vi "main.vi"() -> ()   [LabVIEW 2019]
uses:
  <vilib>/userDefined/High Color/IMAQdx.ctl
  <vilib>/vision/Image Controls.llb/IMAQ Image.ctl
  <vilib>/vision/driver/NI_Vision_Acquisition_Software.lvlib
panel:
  in  "Tab Control":enum32{"Learn Pattern"}(tab)
  in  "Learn":bool
  out "Grab Image Duration":u32
  out "Stop Threads":bool
  out "Grab Running":bool
  out "Image Raw":T1
  out "error out":errorcluster
  in  "Session In":T2
  in  "Snap":bool
  in  "Stop":bool
  in  "Grab":bool
  out "Image Viewer":T1(plugin-control)
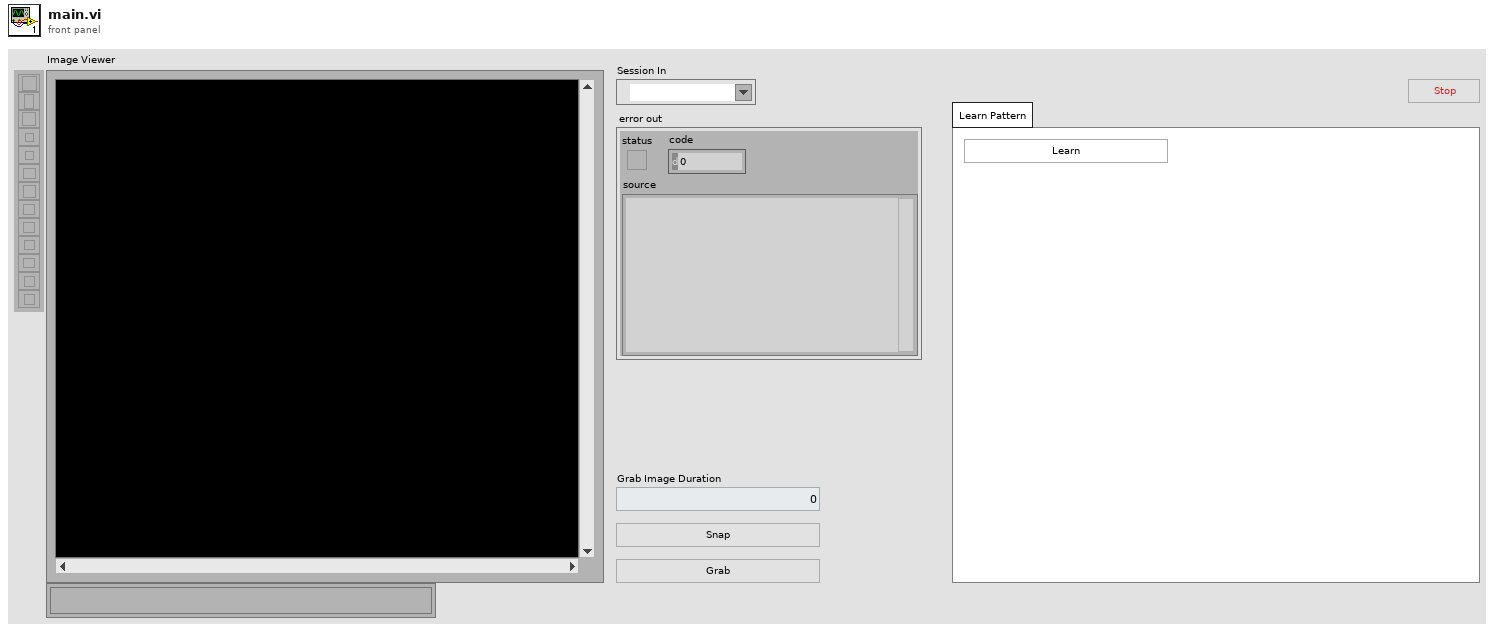
[diagram p1: front panel]
types:
  T1 = typedef "IMAQ Image.ctl" = refnum<image>
  T2 = typedef "IMAQdx.ctl" = refnum<k21>
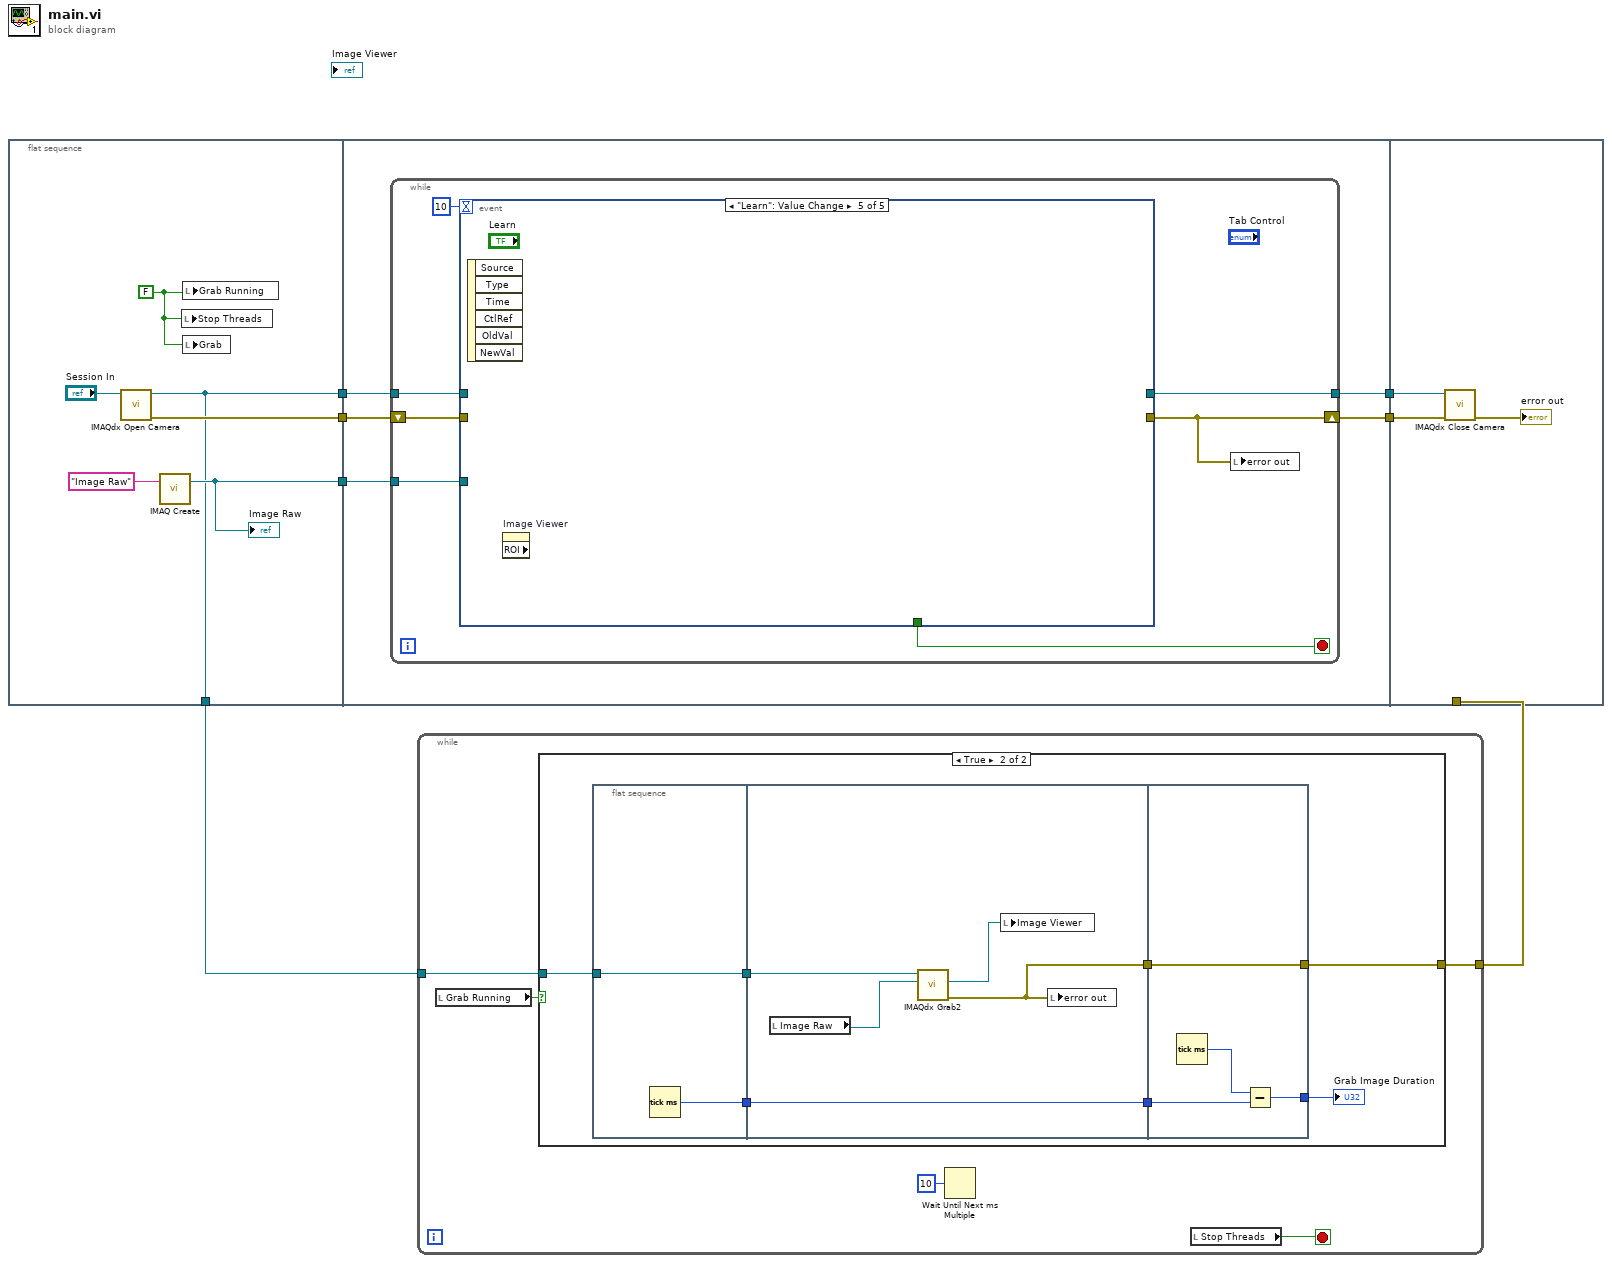
[diagram p0: block diagram]
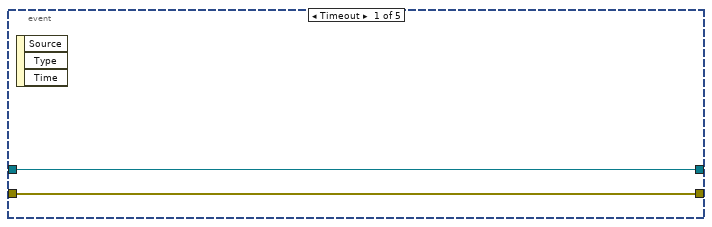
[diagram p3: hidden frame]
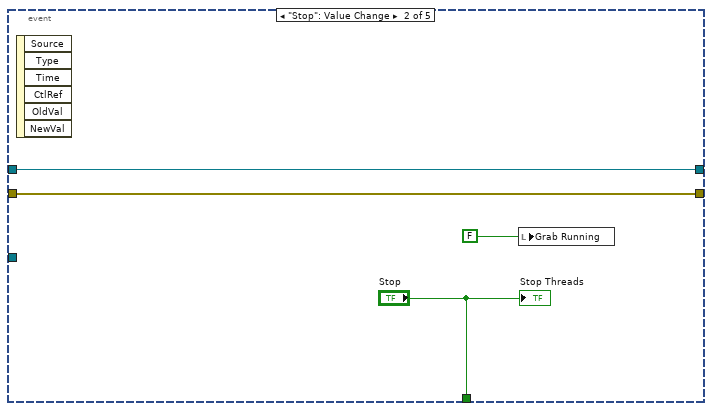
[diagram p4: hidden frame]
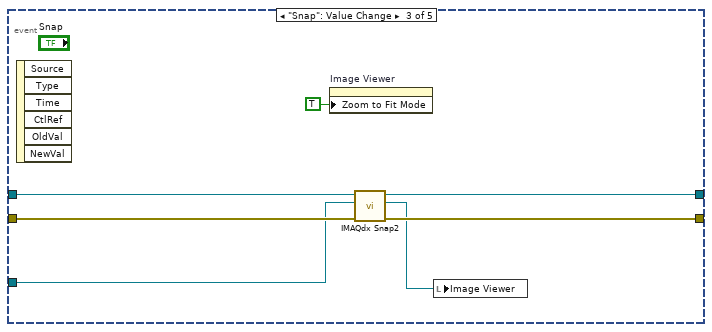
[diagram p5: hidden frame]
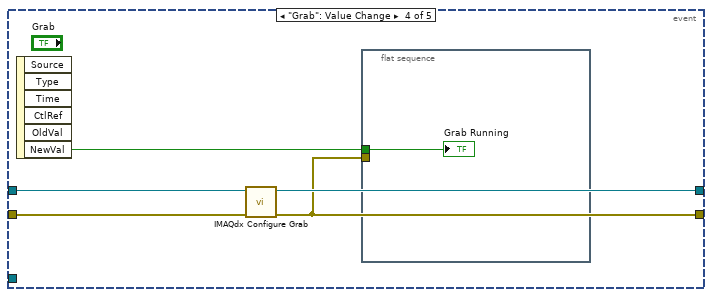
[diagram p6: hidden frame]
diagram:
  n1 = flat-sequence {
    tunnel: [w12] -> w7
    tunnel: [w9] -> w5
    tunnel: [w10] -> w3
    tunnel: [w9] -> w2
    tunnel: w7 -> [w18]
    tunnel: [w17] -> w6
    tunnel: w5 -> [w16]
    tunnel: [w15] -> w4
    tunnel: w3 -> [w14]
    tunnel: w6 -> [w47]
    tunnel: w4 -> [w46]
    tunnel: w1 -> [_]
    frame #0 {
      w8 = FALSE
      n2 = call <vilib>:"IMAQdx Open Camera.vi"("Session In"="Session In") -> ("error out"=w12:errorcluster, "Session Out"=w9:T2)  [unwired: 9 in]
      n3 = call "IMAQ Create"("Image Name"="Image Raw") -> ("New Image"=w10:T1)  [unwired: 4 in, 1 out]
      "Image Raw" <- w10
      n4 = local write "Stop Threads"(w8) -> ()
      n5 = local write "Grab Running"(w8) -> ()
      n6 = local write "Grab"(w8) -> ()
    }
    frame #1 {
      n7 = while {
        shift-right: [w21] -> w17
        shift-left: w18 -> [w22]
        tunnel: w16 -> [w24]
        tunnel: [w23] -> w15
        tunnel: w14 -> [w19]
        stop <- w25 stop-if-true
        n8 = event shown="[4] \"Learn\": Value Change" {
          selector: _ -> [_ _ _ _ _]
          dyn-events: _ -> [_ _ _ _ _]
          timeout: 10 -> [_ _ _ _ _]
          tunnel: [_ "Stop" _ _ _] -> w25
          tunnel: w24 -> [w26 w30 w38 w42 _]
          tunnel: [w26 w30 w36 w40 _] -> w23
          tunnel: w22 -> [w27 w29 w37 w41 _]
          tunnel: [w27 w29 w35 w39 _] -> w21
          tunnel: w19 -> [_ _ w32 _ _]
          event Timeout {
            n9 = event-data() -> ()  [unwired: 1 in, 3 out]
          }
          event "Stop": Value Change {
            n10 = event-data() -> ()  [unwired: 1 in, 6 out]
            n11 = local write "Grab Running"(FALSE ("Grab Running")) -> ()
            "Stop Threads" <- "Stop"
          }
          event "Snap": Value Change {
            n12 = event-data() -> ()  [unwired: 1 in, 6 out]
            n13 = property on="Image Viewer" class="ImageControl"("Zoom to Fit Mode"=TRUE) -> ()  [unwired: 2 in, 2 out]
            n14 = call <vilib>:"IMAQdx Snap2.vi"("error in"=w37, "Image In"=w32, "Session In"=w38) -> ("error out"=w35:errorcluster, "Image Out"=w34:T1, "Session Out"=w36:T2)  [unwired: 6 in]
            n15 = local write "Image Viewer"(w34) -> ()
          }
          event "Grab": Value Change {
            n16 = event-data() -> ("NewVal"=w43:bool)  [unwired: 1 in, 5 out]
            n17 = call <vilib>:"IMAQdx Configure Grab.vi"("error in"=w41, "Session In"=w42) -> ("error out"=w39:errorcluster, "Session Out"=w40:T2)  [unwired: 8 in]
            n18 = flat-sequence {
              tunnel: w43 -> [w44]
              tunnel: w39 -> [_]
              frame #0 {
                "Grab Running" <- w44
              }
            }
          }
          event "Learn": Value Change {
            n19 = event-data() -> ()  [unwired: 1 in, 6 out]
            n20 = property on="Image Viewer" class="ImageControl" props=["ROI"]() -> ()  [unwired: 2 in, 3 out]
          }
        }
        n21 = local write "error out"(w21) -> ()
      }
    }
    frame #2 {
      n22 = call <vilib>:"IMAQdx Close Camera.vi"("error in"=w47, "Session In"=w46) -> ("error out"=→"error out":errorcluster)  [unwired: 9 in]
    }
  }
  n23 = while {
    tunnel: w2 -> [w49]
    tunnel: [w48] -> w1
    stop <- w52 stop-if-true
    n24 = local read "Grab Running"() -> (w51:bool)
    n25 = case shown="True" w51 {
      tunnel: w49 -> [_ w59]
      tunnel: [_ w58] -> w48
      frame False {
      }
      frame True {
        n26 = flat-sequence {
          tunnel: w59 -> [w61]
          tunnel: [w61] -> w57
          tunnel: [w60] -> w55
          tunnel: w57 -> [w64]
          tunnel: [w63] -> w56
          tunnel: w55 -> [w62]
          tunnel: [w62] -> w54
          tunnel: [w70] -> w58
          tunnel: w56 -> [w70]
          tunnel: w54 -> [w69]
          tunnel: [w67] -> w53
          frame #0 {
            n27 = Tick Count (ms)() -> (millisecond timer value=w60:u32)
          }
          frame #1 {
            n28 = local read "Image Raw"() -> (w65:T1)
            n29 = call <vilib>:"IMAQdx Grab2.vi"("Image In"=w65, "Session In"=w64) -> ("error out"=w63:errorcluster, "Image Out"=w66:T1)  [unwired: 6 in, 2 out]
            n30 = local write "Image Viewer"(w66) -> ()
            n31 = local write "error out"(w63) -> ()
          }
          frame #2 {
            n32 = Tick Count (ms)() -> (millisecond timer value=w68:u32)
            n33 = Subtract(x=w68, y=w69) -> (x-y=w67:u32)
          }
        }
        "Grab Image Duration" <- w53
      }
    }
    n34 = Wait Until Next ms Multiple(millisecond multiple=u32 10) -> ()  [unwired: 1 out]
    n35 = local read "Stop Threads"() -> (w52:bool)
  }
